vi "NI-Digital Specific Logic.vi"(8 "error in":errorcluster, 9 "session information":T1, 10 "Measurement Configuration":T5, 11 "instrument handle":refnum<k15>) -> (0 "error out":errorcluster, 2 "Measurement Results":T4, 3 "instrument handle out":refnum<k15>)   [LabVIEW 2020, in "NIDigitalBurstPattern.lvlib"]
uses:
  NIDigitalBurstPattern.lvlib
  Measurement Configuration.ctl
  Measurement Results.ctl
  <vilib>/MeasurementLink/MeasurementLink Session Management Client/RPC Messages/ni_measurementlink_sessionmanagement_v1_SessionInformation.ctl
  <vilib>/MeasurementLink/MeasurementLink Session Management Client/RPC Messages/nidevice_grpc_Session.ctl
  <vilib>/MeasurementLink/MeasurementLink Session Management Client/RPC Messages/ni_measurementlink_sessionmanagement_v1_ChannelMapping.ctl
  <instrlib>/niDigital/niDigital.llb/niDigital Selected Function.ctl
  8a29f827-2a0e-4afd-8fd4-ae2b0b3d3f34.vi
  b0873fce-ae5b-41be-a4cd-e80cfbaeeaa1.vi
  <instrlib>/niDigital/niDigital.llb/niDigital Load Specifications Levels and Timing (Single).vi
  <instrlib>/niDigital/niDigital.llb/niDigital Configure Pattern Label History RAM Trigger.vi
  <instrlib>/niDigital/niDigital.llb/niDigital Burst Pattern (Pass Fail).vi
  <instrlib>/niDigital/niDigital.llb/niDigital Fetch History RAM Cycle Information (1D Pin States).vi
  <vilib>/Comparison/Less/Less Functor/Less Functor.lvclass
  <vilib>/MeasurementLink/MeasurementLink Session Management Client/MeasurementLink Session Management Client.lvlib
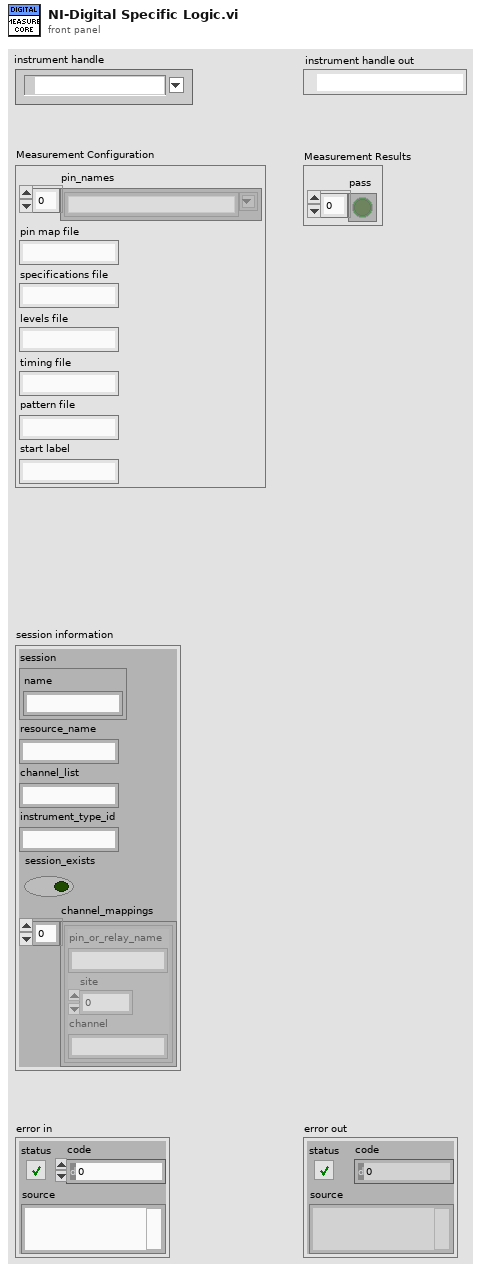
[diagram p1: front panel]
types:
  T1 = typedef "MeasurementLink Session Management Client.lvlib/ni_measurementlink_sessionmanagement_v1_SessionInformation.ctl" = cluster{"session":T2, "resource_name":string, "channel_list":string, "instrument_type_id":string, "session_exists":bool, "channel_mappings":T3[]}
  T2 = typedef "MeasurementLink Session Management Client.lvlib/nidevice_grpc_Session.ctl" = cluster{"name":string}
  T3 = typedef "MeasurementLink Session Management Client.lvlib/ni_measurementlink_sessionmanagement_v1_ChannelMapping.ctl" = cluster{"pin_or_relay_name":string, "site":i32, "channel":string}
  T4 = typedef "NIDigitalBurstPattern.lvlib/Measurement Results.ctl" = cluster{"pass":bool[]}
  T5 = typedef "NIDigitalBurstPattern.lvlib/Measurement Configuration.ctl" = cluster{"pin_names":string[], "pin map file":string, "specifications file":string, "levels file":string, "timing file":string, "pattern file":string, "start label":string}
  T6 = typedef "niDigital Selected Function.ctl" = i32
  T7 = typedef "niDigital History RAM Cycle Information (1D Pin States).ctl" = cluster{"pattern name":string, "time set name":string, "vector number":i64, "cycle number":i64, "expected pin states":T8[], "actual pin states":T8[], "per pin pass fail":bool[]}
  T8 = typedef "niDigital Pin State.ctl" = u8
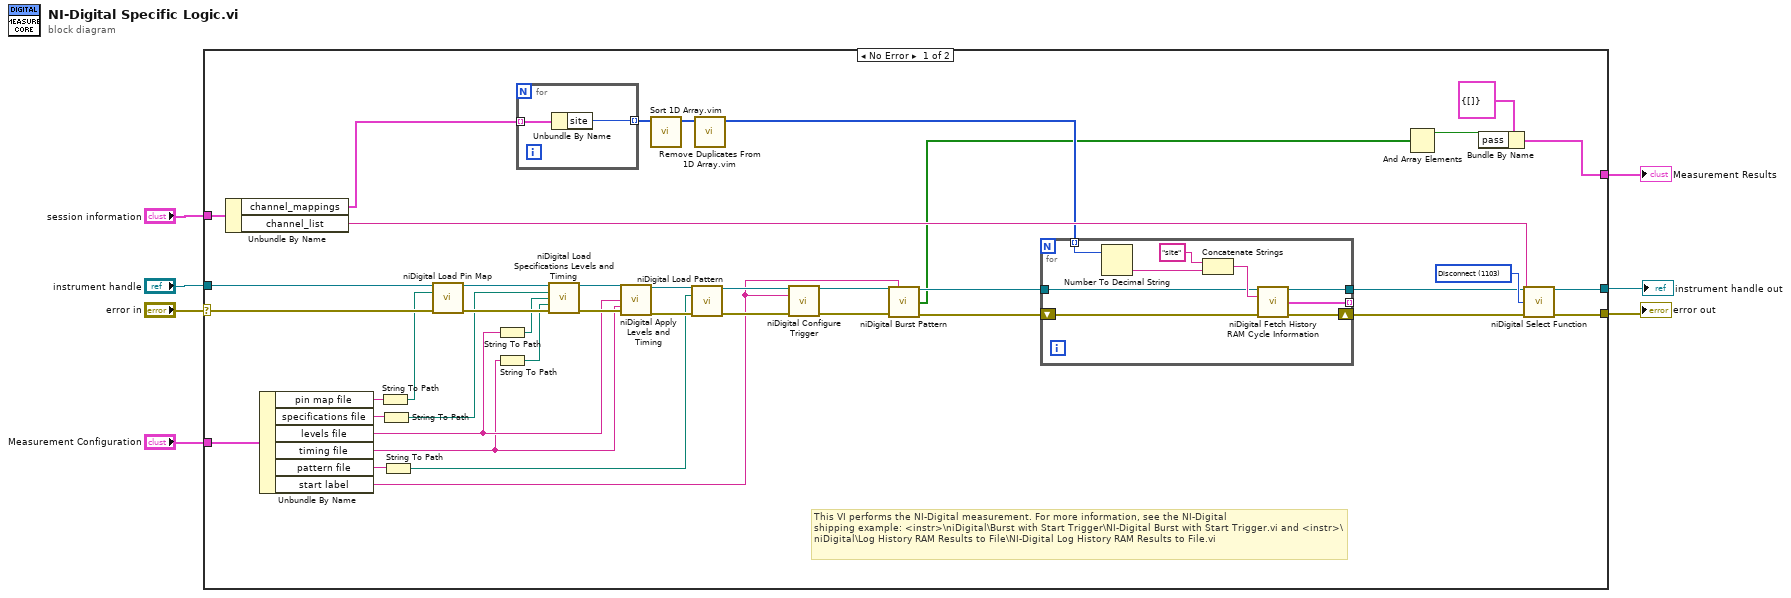
[diagram p0: block diagram]
diagram:
  n1 = case shown="No Error" "error in" {
    selector: "error in" -> [w40 w60]
    tunnel: "Measurement Configuration" -> [w48 _]
    tunnel: [w46 _] -> w6
    tunnel: [w42 w60] -> w5
    tunnel: "instrument handle" -> [w44 w61]
    tunnel: [w43 w61] -> w3
    tunnel: "session information" -> [w45 _]
    frame No Error {
      w41 = T6 1103 items=["Digital"=1100, "PPMU"=1101, "Off"=1102, "Disconnect"=1103] ("function")
      # "This VI performs the NI-Digital measurement. For more information, see the NI-Digital\nshipping example: <instr>\\niDigital\\Burst with Start Trigger\\NI-Digital Burst with Start Trigger.vi and <instr>\\niDigital\\Log History RAM Results to File\\NI-Digital Log History RAM Results to File.vi"
      n2 = Unbundle By Name(w45) -> ("channel_mappings"=w27:T3[], "channel_list"=w28:string)
      n3 = Unbundle By Name(w48) -> ("pin map file"=w17:string, "specifications file"=w15:string, "levels file"=w13:string, "timing file"=w11:string, "pattern file"=w19:string, "start label"=w30:string)
      n4 = String To Path(string=w17) -> (path=w16:path)
      n5 = String To Path(string=w15) -> (path=w14:path)
      n6 = String To Path(string=w19) -> (path=w18:path)
      n7 = call <instrlib>:"niDigital Load Pin Map.vi"("instrument handle"=w44, "pin map file"=w16, "error in"=w40) -> ("instrument handle out"=w38:refnum<k15>, "error out"=w39:errorcluster)  [unwired: 11 in]
      n8 = String To Path(string=w13) -> (path=w12:path)
      n9 = String To Path(string=w11) -> (path=w10:path)
      n10 = for {
        tunnel: w27 -> [w59] mode=indexing
        tunnel: [w58] -> w26 mode=indexing
        n11 = Unbundle By Name(w59) -> ("site"=w58:i32)
      }
      n12 = call-poly <instrlib>:"niDigital Load Specifications Levels and Timing.vi"("instrument handle"=w38, "specifications file path"=w14, "levels file path"=w12, "timing file path"=w10, "error in"=w39) -> ("instrument handle out"=w36:refnum<k15>, "error out"=w37:errorcluster)  [unwired: 9 in]
      n13 = call <instrlib>:"niDigital Apply Levels and Timing.vi"("instrument handle"=w36, "levels sheet"=w13, "timing sheet"=w11, "error in"=w37) -> ("instrument handle out"=w34:refnum<k15>, "error out"=w35:errorcluster)  [unwired: 10 in]
      n14 = call "Sort 1D Array.vim"("unsorted array"=w26) -> ("sorted array"=w25:i32[])  [unwired: 10 in]
      n15 = call <instrlib>:"niDigital Load Pattern.vi"("instrument handle"=w34, "pattern file"=w18, "error in"=w35) -> ("instrument handle out"=w33:refnum<k15>, "error out"=w31:errorcluster)  [unwired: 11 in]
      n16 = call "Remove Duplicates From 1D Array.vim"("array"=w25) -> ("array with duplicates removed"=w24:i32[])  [unwired: 10 in]
      n17 = call-poly <instrlib>:"niDigital Configure Trigger.vi"("instrument handle"=w33, "label"=w30, "error in"=w31) -> ("instrument handle out"=w32:refnum<k15>, "error out"=w29:errorcluster)  [unwired: 11 in]
      n18 = call-poly <instrlib>:"niDigital Burst Pattern.vi"("instrument handle"=w32, "start label"=w30, "error in"=w29) -> ("instrument handle out"=w20:refnum<k15>, "pass"=w9:bool[], "error out"=w23:errorcluster)  [unwired: 10 in]
      n19 = for {
        tunnel: w24 -> [w52] mode=indexing
        shift-right: [w56] -> w22
        shift-left: w23 -> [w57]
        tunnel: [w55] -> w21
        tunnel: w20 -> [w50]
        tunnel: [w49] -> _ mode=indexing
        n20 = Number To Decimal String(number=w52) -> (decimal integer string=w53:string)  [unwired: 1 in]
        n21 = Concatenate Strings("site" ("string"), w53) -> (w51:string)
        n22 = call-poly <instrlib>:"niDigital Fetch History RAM Cycle Information.vi"("instrument handle"=w50, "site"=w51, "error in"=w57) -> ("instrument handle out"=w55:refnum<k15>, "cycle information"=w49:T7[], "error out"=w56:errorcluster)  [unwired: 10 in]
      }
      n23 = And Array Elements(Boolean array=w9) -> (logical AND=w8:bool)
      n24 = Bundle By Name(cluster=T4 {"pass"=[]} ("Measurement Results"), "pass"=w8) -> (w46:T4)
      n25 = call <instrlib>:"niDigital Select Function.vi"("instrument handle"=w21, "channel list"=w28, "function"=w41, "error in"=w22) -> ("instrument handle out"=w43:refnum<k15>, "error out"=w42:errorcluster)  [unwired: 10 in]
    }
    frame Error {
    }
  }
  "Measurement Results" <- w6
  "error out" <- w5
  "instrument handle out" <- w3
